vi "Read Output Scale Factor (V_degrees).vi"(8 "error in (no error)":errorcluster, 11 "Galvonometer in":refnum<class "Galvonometer.lvclass">) -> (0 "error out":errorcluster, 2 "Output Scale Factor (V/degrees)":dbl=0.5, 3 "Galvonometer out":refnum<class "Galvonometer.lvclass">)   [LabVIEW 2017, in "Galvonometer.lvclass"]
uses:
  Galvonometer.lvclass
  Galvonometer.lvclass/Galvonometer.ctl
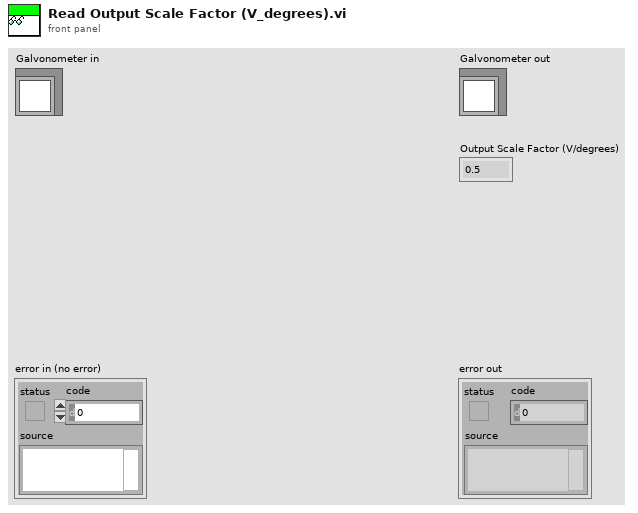
[diagram p1: front panel]
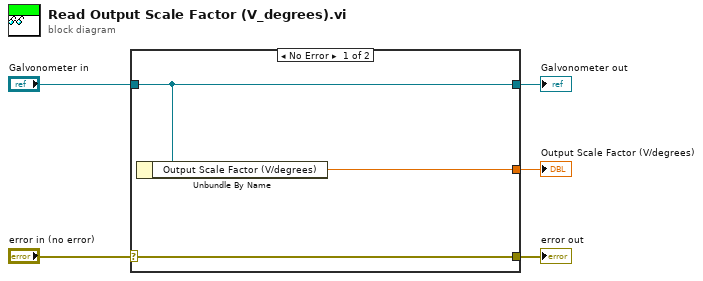
[diagram p0: block diagram]
diagram:
  n1 = case shown="No Error" "error in (no error)" {
    selector: "error in (no error)" -> [w8 w9]
    tunnel: [w8 w9] -> w4
    tunnel: [w7 w10] -> w2
    tunnel: "Galvonometer in" -> [w7 w10]
    tunnel: [w6 _] -> w1
    frame No Error {
      n2 = Unbundle By Name(w7) -> ("Output Scale Factor (V/degrees)"=w6:dbl)
    }
    frame Error {
    }
  }
  "error out" <- w4
  "Galvonometer out" <- w2
  "Output Scale Factor (V/degrees)" <- w1
